vi "Logger Ready.vi"(8 "error in (no error)":errorcluster, 10 "Logger Ready":T1, 11 "Log Manager Module in":refnum<class "Log Manager Module.lvclass">) -> (0 "error out":errorcluster, 3 "Log Manager Module out":refnum<class "Log Manager Module.lvclass">)   [LabVIEW 2020, in "VolatusData.lvlib" / "Log Manager Module.lvclass"]
uses:
  Log Manager Module.lvclass
  C:/dev/lv20CE/relink/lv-volatus/Volatus/Module/Module.lvclass
  Logger Ready.ctl
  Log Manager Module.lvclass/Log Manager Module.ctl
  Logger State.ctl
  Volatus/Module/Module.lvclass/Module.ctl
  Volatus/Event Level.ctl
  Volatus/Module/Module.lvclass
  VolatusData.lvlib
  Volatus/Volatus.lvlib
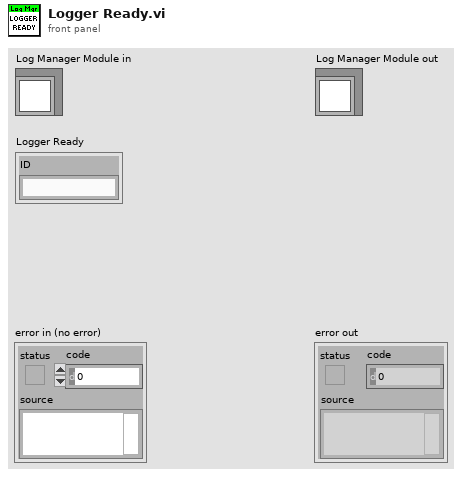
[diagram p1: front panel]
types:
  T1 = typedef "VolatusData.lvlib/Logger Ready.ctl" = cluster{"ID":string}
  T2 = typedef "VolatusData.lvlib/Logger State.ctl" = enum16{"Unknown", "Idle", "Preparing", "Ready", "Logging", "Stopping"}
  T3 = typedef "VolatusData.lvlib/Log Manager Module.lvclass/Group Info.ctl" = cluster{"Name":string, "Loggers":map{string, T4}}
  T4 = typedef "VolatusData.lvlib/Log Manager Module.lvclass/Logger.ctl" = cluster{"ID":string, "MsgQ":refnum<class "MessageQ.lvclass">, "State":T2, "Group":string}
  T5 = typedef "Volatus.lvlib/Event Level.ctl" = enum16{"Debug", "Info", "Warning", "Error"}
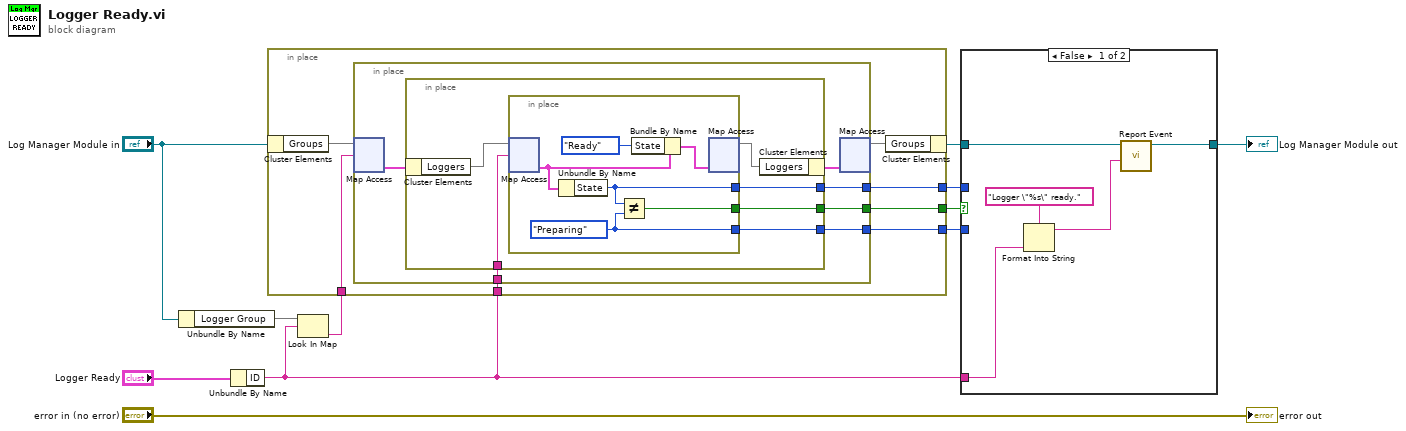
[diagram p0: block diagram]
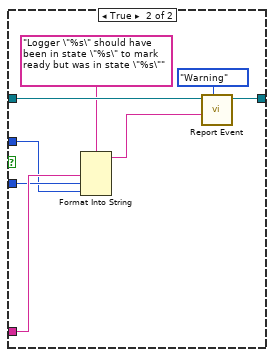
[diagram p2: hidden frame]
diagram:
  n1 = Unbundle By Name("Log Manager Module in") -> ("Logger Group"=w3:map{string, string})
  n2 = Unbundle By Name("Logger Ready") -> ("ID"=w2:string)
  n3 = Look In Map(map=w3, key=w2) -> (value=w1:string)  [unwired: 1 in, 1 out]
  n4 = in-place {
    in-place-border: [w18] -> w8
    in-place-border: [w17] -> w7
    in-place-border: [w16] -> w6
    in-place-border: w2 -> [w15]
    in-place-border: w1 -> [w13]
    n5 = in-place-cluster #1("Log Manager Module in") -> ("Groups"=w14:map{string, T3})
    n6 = in-place {
      in-place-border: [w24] -> w18
      in-place-border: [w23] -> w17
      in-place-border: [w22] -> w16
      in-place-border: w15 -> [w21]
      n7 = in-place-map #2(w14, w13) -> (w20:T3)  [unwired: 1 in, 1 out]
      n8 = in-place {
        in-place-border: [w30] -> w24
        in-place-border: [w29] -> w23
        in-place-border: [w28] -> w22
        in-place-border: w21 -> [w27]
        n9 = in-place-cluster #3(w20) -> ("Loggers"=w26:map{string, T4})
        n10 = in-place {
          in-place-border: [w33] -> w30
          in-place-border: [w32] -> w29
          in-place-border: [w31] -> w28
          w31 = Logger_State."Preparing" ("y")
          n11 = in-place-map #4(w26, w27) -> (w36:T4)  [unwired: 1 in, 1 out]
          n12 = Unbundle By Name(w36) -> ("State"=w32:T2)
          n13 = Not Equal?(x=w32, y=w31) -> (x != y?=w33:bool)
          n14 = Bundle By Name(cluster=w36, "State"=Logger_State."Ready") -> (w34:T4)
          n15 = in-place-map #4(w34) -> (w25:map{string, T4})  [unwired: 1 in, 2 out]
        }
        n16 = in-place-cluster #3("Loggers"=w25) -> (w19:T3)
      }
      n17 = in-place-map #2(w19) -> (w12:map{string, T3})  [unwired: 1 in, 2 out]
    }
    n18 = in-place-cluster #1("Groups"=w12) -> (w9:refnum<class "Log Manager Module.lvclass">)
  }
  n19 = case shown="False" w8 {
    tunnel: w9 -> [w41 w49]
    tunnel: w7 -> [_ w44]
    tunnel: w6 -> [_ w45]
    tunnel: w2 -> [w38 w46]
    tunnel: [w40 w42] -> w5
    frame False {
      n20 = Format Into String(format string="Logger \"%s\" ready.", w38) -> (resulting string=w37:string)  [unwired: 2 in, 1 out]
      n21 = call "Report Event.vi"("Message"=w37, "Module in"=w41) -> ("Module out"=w40:refnum<class "Log Manager Module.lvclass">)  [unwired: 8 in, 1 out]
    }
    frame True {
      n22 = Format Into String(format string="Logger \"%s\" should have been in state \"%s\" to mark ready but was in state \"%s\"", w46, w45, w44) -> (resulting string=w43:string)  [unwired: 2 in, 1 out]
      n23 = call "Report Event.vi"("Level (Info)"=Event_Level."Warning", "Message"=w43, "Module in"=w49) -> ("Module out"=w42:refnum<class "Log Manager Module.lvclass">)  [unwired: 7 in, 1 out]
    }
  }
  "Log Manager Module out" <- w5
  "error out" <- "error in (no error)"
